vi "Lab Panel V4.91.vi"() -> ()   [LabVIEW 2013] (continued)
                                (unwired) FALSE
                                n567 = String To Path(string=w889) -> (path=w885:path)
                                n568 = TDMS Open(6:FALSE, 10:T20."create or replace" ("operation (0:open)"), 11:w885) -> (0:w884:errorcluster, 3:→"TDMS LAB01-2":refnum<k34>)  [unwired: 4 in]
                              }
                              frame #2 {
                                n569 = local read "SET LAB01-2"() -> (w895:T5)
                                n570 = local read "TDMS LAB01-2"() -> (w906:refnum<k34>)
                                n571 = Build Array("Testers Name", "Description", "Set Test Cycles", "T-Rise minutes", "T-Rise Deg C") -> (w896:string[])
                                n572 = Unbundle(w895) -> ("NAME"=w894:string, "DESCRIPTION"=w893:string, "CYCLES"=w892:dbl, "T-RISE mins"=w891:dbl, "T-RISE deg C"=w890:dbl)
                                n573 = Number To Decimal String(number=w892) -> (decimal integer string=w905:string)  [unwired: 1 in]
                                n574 = Number To Decimal String(number=w891) -> (decimal integer string=w904:string)  [unwired: 1 in]
                                n575 = Number To Decimal String(number=w890) -> (decimal integer string=w903:string)  [unwired: 1 in]
                                n576 = Build Array(w894, w893, w905, w904, w903) -> (w902:string[])
                                n577 = TDMS Set Properties(5:w902, 7:w896, 11:w906) -> ()  [unwired: 3 in, 4 out]
                              }
                              frame #3 {
                                n578 = local read "DISP LAB01-2"() -> (w908:T4)
                                n579 = Concatenate Strings("LAB01-2  ", w911) -> (w912:string)
                                n580 = Two Button Dialog(message=w912, 1:w909, 2:w910) -> (T button?=w914:bool)
                                n581 = case shown="True" w914 {
                                tunnel: w908 -> [w921 w922]
                                tunnel: [w921 w922] -> w918
                                tunnel: [w920 w923] -> w917
                                tunnel: [w919 w923] -> w916
                                frame False {
                                n582 = Unbundle(w921) -> ("CYCLE"=w920:dbl, "MINS"=w919:dbl)  [unwired: 1 out]
                                }
                                frame True {
                                w923 = 0.0
                                }
                                }
                                n583 = Bundle(cluster=w918, "CYCLE"=w917, "MINS"=w916, "STATUS"="RUN") -> (w907:T4)
                                n584 = local write "DISP LAB01-2"(w907) -> ()
                              }
                              frame #4 {
                                n585 = local read "TEMP START LAB01-2"() -> (w926:cluster{"TL":dbl, "TN":dbl})
                                n586 = Bundle(cluster=w926, "TL"=w924, "TN"=w924) -> (w925:cluster{"TL":dbl, "TN":dbl})
                                n587 = local write "TEMP START LAB01-2"(w925) -> ()
                              }
                            }
                          }
                        }
                      }
                    }
                  }
                }
              }
              event "RUN LAB02-1": Value Change {
                n588 = event-data() -> ("NewVal"=w932:bool)  [unwired: 1 in, 5 out]
                n589 = local read "SIG LAB02-1"() -> (w928:T2)
                n590 = case shown="True" w932 {
                  tunnel: w938 -> [_ w976]
                  tunnel: w937 -> [_ w975]
                  tunnel: w935 -> [w940 w974]
                  tunnel: w936 -> [_ w973]
                  tunnel: w934 -> [_ w972]
                  tunnel: [w939 w971] -> w933
                  tunnel: w931 -> [_ w970]
                  tunnel: w930 -> [_ w969]
                  tunnel: w929 -> [_ w968]
                  tunnel: w928 -> [_ w967]
                  tunnel: w927 -> [_ w966]
                  frame False {
                    # "stop test"
                    n591 = stacked-sequence {
                      tunnel: w940 -> [w949 _]
                      tunnel: [w941 _] -> w939
                      frame #0 {
                        n592 = local read "DISP LAB02-1"() -> (w948:T4)
                        n593 = Unbundle(w948) -> ("CYCLE"=w946:dbl, "MINS"=w947:dbl)  [unwired: 1 out]
                        n594 = case shown="\"CYCLE TEST\"" w949 {
                          tunnel: w947 -> [_ _ w956]
                          tunnel: w946 -> [w954 w955 _]
                          tunnel: [w954 w955 w956] -> w945
                          frame "CHART TEST", Default {
                          }
                          frame "CYCLE TEST" {
                          }
                          frame "T-RISE TEST" {
                          }
                        }
                        n595 = local read "TDMS LAB02-1"() -> (w953:refnum<k34>)
                        n596 = Build Array("STOPPED") -> (w950:string[])
                        n597 = Build Array(w945) -> (w944:dbl[])
                        n598 = TDMS Write(0:w953, 5:"TEST RESULT", 7:w950, 9:w944) -> (4:w942:refnum<k34>, 15:w943:errorcluster)  [unwired: 2 in, 2 out]
                        n599 = TDMS Close(8:w943, 11:w942) -> (0:w941:errorcluster)  [unwired: 1 out]
                      }
                      frame #1 {
                        n600 = local read "DISP LAB02-1"() -> (w960:T4)
                        n601 = stacked-sequence {
                          tunnel: "LAB02-1" -> [w962 w964]
                          frame #0 {
                            n602 = call "sub vi - defrag tdms v1.vi"("panel id"=w962) -> ("error out"=w961:errorcluster)  [unwired: 10 in]
                            n603 = local write "data file error"(w961) -> ()
                          }
                          frame #1 {
                            n604 = local write "RESULT LAB02-1"(FALSE) -> ()
                            n605 = call "Save data file (stop) v3.vi"("panel id"=w964) -> ("network file save error"=w963:errorcluster)  [unwired: 9 in, 1 out]
                            n606 = local write "data file error"(w963) -> ()
                          }
                        }
                        n607 = Bundle(cluster=w960, "STATUS"="STOP") -> (w958:T4)  [unwired: 2 in]
                        n608 = local write "DISP LAB02-1"(w958) -> ()
                      }
                    }
                  }
                  frame True {
                    n609 = stacked-sequence {
                      seq-local: [w978 _] -> [_ w982]
                      tunnel: w976 -> [_ w992]
                      tunnel: w975 -> [_ w991]
                      tunnel: w974 -> [_ w990]
                      tunnel: w973 -> [_ w989]
                      tunnel: w972 -> [_ w988]
                      tunnel: [_ w987] -> w971
                      tunnel: w970 -> [_ w986]
                      tunnel: w969 -> [_ w985]
                      tunnel: w968 -> [_ w984]
                      tunnel: w967 -> [w977 w983]
                      tunnel: w966 -> [_ w981]
                      frame #0 {
                        n610 = Unbundle(w977) -> ("AMPS"=w980:dbl)  [unwired: 4 out]
                        n611 = call "Check For Amps on v1.vi"("ID"="LAB02-1", "amps"=w980) -> ("amps"=w978:bool)  [unwired: 9 in]
                      }
                      frame #1 {
                        n612 = case shown="True" w982 {
                          tunnel: w992 -> [_ w1005]
                          tunnel: w991 -> [_ w1004]
                          tunnel: w990 -> [_ w1003]
                          tunnel: w989 -> [_ w1002]
                          tunnel: w988 -> [_ w1001]
                          tunnel: [errorcluster {"status"=FALSE, "code"=0, "source"=""} ("error out") w1000] -> w987
                          tunnel: w986 -> [_ w999]
                          tunnel: w985 -> [_ w998]
                          tunnel: w984 -> [_ w997]
                          tunnel: w983 -> [_ w996]
                          tunnel: w981 -> [_ w995]
                          frame False {
                            w994 = FALSE
                            n613 = local write "RUN LAB02-1"(w994) -> ()
                            n614 = local write "run lab02-1"(w994) -> ()
                          }
                          frame True {
                            n615 = stacked-sequence {
                              seq-local: [w1006 _ _ _ _] -> [_ w1030 _ _ _]
                              tunnel: w1005 -> [w1011 _ _ _ _]
                              tunnel: w1004 -> [w1008 _ _ _ _]
                              tunnel: w1003 -> [w1021 _ _ _ _]
                              tunnel: w1002 -> [w1014 _ _ _ _]
                              tunnel: w1001 -> [w1009 _ _ _ _]
                              tunnel: [_ w1025 _ _ _] -> w1000
                              tunnel: w999 -> [_ _ _ w1051 _]
                              tunnel: w998 -> [_ _ _ w1050 _]
                              tunnel: w997 -> [_ _ _ w1049 _]
                              tunnel: w996 -> [_ _ _ _ _]
                              tunnel: w995 -> [_ _ _ _ w1065]
                              frame #0 {
                                w1007 = "\\"
                                n616 = local read "SET LAB02-1"() -> (w1016:T5)
                                n617 = case shown="\"CYCLE TEST\"" w1021 {
                                tunnel: ["L02-1-CHART TEST-" "L02-1-CYCLE TEST-" "L02-1-T-RISE TEST-"] -> w1017
                                frame "CHART TEST", Default {
                                }
                                frame "CYCLE TEST" {
                                }
                                frame "T-RISE TEST" {
                                }
                                }
                                n618 = Unbundle(w1016) -> ("DESCRIPTION"=w1015:string)  [unwired: 4 out]
                                n619 = Concatenate Strings(w1011, "\\", w1009, w1007, w1008, w1007) -> (w1018:string)
                                n620 = String To Path(string=w1018) -> (path=w1020:path)
                                n621 = Concatenate Strings(w1018, w1017, w1015, "-", w1014, ".tdms") -> (w1006:string)
                                n622 = Create Folder(path (use dialog)=w1020) -> (error out=w1019:errorcluster)  [unwired: 2 in, 2 out]
                                n623 = global write "Global 1.vi" "LAB02-1 FILE"(w1006) -> ()
                                n624 = call <vilib>:"Clear Errors.vi"("error in (no error)"=w1019) -> ()  [unwired: 6 in, 1 out]
                              }
                              frame #1 {
                                (unwired) FALSE
                                n625 = String To Path(string=w1030) -> (path=w1026:path)
                                n626 = TDMS Open(6:FALSE, 10:T20."create or replace" ("operation (0:open)"), 11:w1026) -> (0:w1025:errorcluster, 3:→"TDMS LAB02-1":refnum<k34>)  [unwired: 4 in]
                              }
                              frame #2 {
                                n627 = local read "SET LAB02-1"() -> (w1036:T5)
                                n628 = local read "TDMS LAB02-1"() -> (w1047:refnum<k34>)
                                n629 = Build Array("Testers Name", "Description", "Set Test Cycles", "T-Rise minutes", "T-Rise Deg C") -> (w1037:string[])
                                n630 = Unbundle(w1036) -> ("NAME"=w1035:string, "DESCRIPTION"=w1034:string, "CYCLES"=w1033:dbl, "T-RISE mins"=w1032:dbl, "T-RISE deg C"=w1031:dbl)
                                n631 = Number To Decimal String(number=w1033) -> (decimal integer string=w1046:string)  [unwired: 1 in]
                                n632 = Number To Decimal String(number=w1032) -> (decimal integer string=w1045:string)  [unwired: 1 in]
                                n633 = Number To Decimal String(number=w1031) -> (decimal integer string=w1044:string)  [unwired: 1 in]
                                n634 = Build Array(w1035, w1034, w1046, w1045, w1044) -> (w1043:string[])
                                n635 = TDMS Set Properties(5:w1043, 7:w1037, 11:w1047) -> ()  [unwired: 3 in, 4 out]
                              }
                              frame #3 {
                                n636 = local read "DISP LAB02-1"() -> (w1052:T4)
                                n637 = Concatenate Strings("LAB02-1  ", w1051) -> (w1053:string)
                                n638 = Two Button Dialog(message=w1053, 1:w1049, 2:w1050) -> (T button?=w1055:bool)
                                n639 = case shown="True" w1055 {
                                tunnel: w1052 -> [w1062 w1063]
                                tunnel: [w1062 w1063] -> w1059
                                tunnel: [w1061 w1064] -> w1058
                                tunnel: [w1060 w1064] -> w1057
                                frame False {
                                n640 = Unbundle(w1062) -> ("CYCLE"=w1061:dbl, "MINS"=w1060:dbl)  [unwired: 1 out]
                                }
                                frame True {
                                w1064 = 0.0
                                }
                                }
                                n641 = Bundle(cluster=w1059, "CYCLE"=w1058, "MINS"=w1057, "STATUS"="RUN") -> (w1048:T4)
                                n642 = local write "DISP LAB02-1"(w1048) -> ()
                              }
                              frame #4 {
                                n643 = local read "TEMP START LAB02-1"() -> (w1067:cluster{"TL":dbl, "TN":dbl})
                                n644 = Bundle(cluster=w1067, "TL"=w1065, "TN"=w1065) -> (w1066:cluster{"TL":dbl, "TN":dbl})
                                n645 = local write "TEMP START LAB02-1"(w1066) -> ()
                              }
                            }
                          }
                        }
                      }
                    }
                  }
                }
                n646 = local write "run lab02-1"(w932) -> ()
              }
              event "RUN LAB02-2": Value Change {
                n647 = event-data() -> ("NewVal"=w1072:bool)  [unwired: 1 in, 5 out]
                n648 = local write "run lab02-2"(w1072) -> ()
                n649 = case shown="True" w1072 {
                  tunnel: w1078 -> [_ w1116]
                  tunnel: w1077 -> [_ w1115]
                  tunnel: w1075 -> [w1080 w1114]
                  tunnel: w1076 -> [_ w1113]
                  tunnel: w1074 -> [_ w1112]
                  tunnel: [w1079 w1111] -> w1073
                  tunnel: w1071 -> [_ w1110]
                  tunnel: w1070 -> [_ w1109]
                  tunnel: w1069 -> [_ w1108]
                  tunnel: w1068 -> [_ w1106]
                  frame False {
                    # "stop test"
                    n650 = stacked-sequence {
                      tunnel: w1080 -> [w1089 _]
                      tunnel: [w1081 _] -> w1079
                      frame #0 {
                        n651 = local read "DISP LAB02-2"() -> (w1088:T4)
                        n652 = Unbundle(w1088) -> ("CYCLE"=w1086:dbl, "MINS"=w1087:dbl)  [unwired: 1 out]
                        n653 = case shown="\"CYCLE TEST\"" w1089 {
                          tunnel: w1087 -> [_ _ w1096]
                          tunnel: w1086 -> [w1094 w1095 _]
                          tunnel: [w1094 w1095 w1096] -> w1085
                          frame "CHART TEST", Default {
                          }
                          frame "CYCLE TEST" {
                          }
                          frame "T-RISE TEST" {
                          }
                        }
                        n654 = local read "TDMS LAB02-2"() -> (w1093:refnum<k34>)
                        n655 = Build Array("STOPPED") -> (w1090:string[])
                        n656 = Build Array(w1085) -> (w1084:dbl[])
                        n657 = TDMS Write(0:w1093, 5:"TEST RESULT", 7:w1090, 9:w1084) -> (4:w1082:refnum<k34>, 15:w1083:errorcluster)  [unwired: 2 in, 2 out]
                        n658 = TDMS Close(8:w1083, 11:w1082) -> (0:w1081:errorcluster)  [unwired: 1 out]
                      }
                      frame #1 {
                        n659 = local read "DISP LAB02-2"() -> (w1100:T4)
                        n660 = stacked-sequence {
                          tunnel: "LAB02-2" -> [w1102 w1104]
                          frame #0 {
                            n661 = call "sub vi - defrag tdms v1.vi"("panel id"=w1102) -> ("error out"=w1101:errorcluster)  [unwired: 10 in]
                            n662 = local write "data file error"(w1101) -> ()
                          }
                          frame #1 {
                            n663 = call "Save data file (stop) v3.vi"("panel id"=w1104) -> ("network file save error"=w1103:errorcluster)  [unwired: 9 in, 1 out]
                            n664 = local write "RESULT LAB02-2"(FALSE) -> ()
                            n665 = local write "data file error"(w1103) -> ()
                          }
                        }
                        n666 = Bundle(cluster=w1100, "STATUS"="STOP") -> (w1098:T4)  [unwired: 2 in]
                        n667 = local write "DISP LAB02-2"(w1098) -> ()
                      }
                    }
                  }
                  frame True {
                    n668 = local read "SIG LAB02-2"() -> (w1107:T2)
                    n669 = stacked-sequence {
                      seq-local: [w1118 _] -> [_ w1122]
                      tunnel: w1116 -> [_ w1132]
                      tunnel: w1115 -> [_ w1131]
                      tunnel: w1114 -> [_ w1130]
                      tunnel: w1113 -> [_ w1129]
                      tunnel: w1112 -> [_ w1128]
                      tunnel: [_ w1127] -> w1111
                      tunnel: w1110 -> [_ w1126]
                      tunnel: w1109 -> [_ w1125]
                      tunnel: w1108 -> [_ w1124]
                      tunnel: w1107 -> [w1117 w1123]
                      tunnel: w1106 -> [_ w1121]
                      frame #0 {
                        n670 = Unbundle(w1117) -> ("AMPS"=w1120:dbl)  [unwired: 4 out]
                        n671 = call "Check For Amps on v1.vi"("ID"="LAB02-2", "amps"=w1120) -> ("amps"=w1118:bool)  [unwired: 9 in]
                      }
                      frame #1 {
                        n672 = case shown="True" w1122 {
                          tunnel: w1132 -> [_ w1145]
                          tunnel: w1131 -> [_ w1144]
                          tunnel: w1130 -> [_ w1143]
                          tunnel: w1129 -> [_ w1142]
                          tunnel: w1128 -> [_ w1141]
                          tunnel: [errorcluster {"status"=FALSE, "code"=0, "source"=""} ("error out") w1140] -> w1127
                          tunnel: w1126 -> [_ w1139]
                          tunnel: w1125 -> [_ w1138]
                          tunnel: w1124 -> [_ w1137]
                          tunnel: w1123 -> [_ w1136]
                          tunnel: w1121 -> [_ w1135]
                          frame False {
                            w1133 = FALSE
                            n673 = local write "RUN LAB02-2"(w1133) -> ()
                            n674 = local write "run lab02-2"(w1133) -> ()
                          }
                          frame True {
                            n675 = stacked-sequence {
                              seq-local: [w1146 _ _ _ _] -> [_ w1170 _ _ _]
                              tunnel: w1145 -> [w1151 _ _ _ _]
                              tunnel: w1144 -> [w1148 _ _ _ _]
                              tunnel: w1143 -> [w1161 _ _ _ _]
                              tunnel: w1142 -> [w1154 _ _ _ _]
                              tunnel: w1141 -> [w1149 _ _ _ _]
                              tunnel: [_ w1165 _ _ _] -> w1140
                              tunnel: w1139 -> [_ _ _ w1191 _]
                              tunnel: w1138 -> [_ _ _ w1190 _]
                              tunnel: w1137 -> [_ _ _ w1189 _]
                              tunnel: w1136 -> [_ _ _ _ _]
                              tunnel: w1135 -> [_ _ _ _ w1205]
                              frame #0 {
                                w1147 = "\\"
                                n676 = local read "SET LAB02-2"() -> (w1156:T5)
                                n677 = case shown="\"CYCLE TEST\"" w1161 {
                                tunnel: ["L02-2-CHART TEST-" "L02-2-CYCLE TEST-" "L02-2-T-RISE TEST-"] -> w1157
                                frame "CHART TEST", Default {
                                }
                                frame "CYCLE TEST" {
                                }
                                frame "T-RISE TEST" {
                                }
                                }
                                n678 = Unbundle(w1156) -> ("DESCRIPTION"=w1155:string)  [unwired: 4 out]
                                n679 = Concatenate Strings(w1151, "\\", w1149, w1147, w1148, w1147) -> (w1158:string)
                                n680 = String To Path(string=w1158) -> (path=w1160:path)
                                n681 = Concatenate Strings(w1158, w1157, w1155, "-", w1154, ".tdms") -> (w1146:string)
                                n682 = Create Folder(path (use dialog)=w1160) -> (error out=w1159:errorcluster)  [unwired: 2 in, 2 out]
                                n683 = global write "Global 1.vi" "LAB02-2 FILE"(w1146) -> ()
                                n684 = call <vilib>:"Clear Errors.vi"("error in (no error)"=w1159) -> ()  [unwired: 6 in, 1 out]
                              }
                              frame #1 {
                                (unwired) FALSE
                                n685 = String To Path(string=w1170) -> (path=w1166:path)
                                n686 = TDMS Open(6:FALSE, 10:T20."create or replace" ("operation (0:open)"), 11:w1166) -> (0:w1165:errorcluster, 3:→"TDMS LAB02-2":refnum<k34>)  [unwired: 4 in]
                              }
                              frame #2 {
                                n687 = local read "SET LAB02-2"() -> (w1176:T5)
                                n688 = local read "TDMS LAB02-2"() -> (w1187:refnum<k34>)
                                n689 = Build Array("Testers Name", "Description", "Set Test Cycles", "T-Rise minutes", "T-Rise Deg C") -> (w1177:string[])
                                n690 = Unbundle(w1176) -> ("NAME"=w1175:string, "DESCRIPTION"=w1174:string, "CYCLES"=w1173:dbl, "T-RISE mins"=w1172:dbl, "T-RISE deg C"=w1171:dbl)
                                n691 = Number To Decimal String(number=w1173) -> (decimal integer string=w1186:string)  [unwired: 1 in]
                                n692 = Number To Decimal String(number=w1172) -> (decimal integer string=w1185:string)  [unwired: 1 in]
                                n693 = Number To Decimal String(number=w1171) -> (decimal integer string=w1184:string)  [unwired: 1 in]
                                n694 = Build Array(w1175, w1174, w1186, w1185, w1184) -> (w1183:string[])
                                n695 = TDMS Set Properties(5:w1183, 7:w1177, 11:w1187) -> ()  [unwired: 3 in, 4 out]
                              }
                              frame #3 {
                                n696 = local read "DISP LAB02-2"() -> (w1192:T4)
                                n697 = Concatenate Strings("LAB02-2  ", w1191) -> (w1193:string)
                                n698 = Two Button Dialog(message=w1193, 1:w1189, 2:w1190) -> (T button?=w1195:bool)
                                n699 = case shown="True" w1195 {
                                tunnel: w1192 -> [w1202 w1203]
                                tunnel: [w1202 w1203] -> w1199
                                tunnel: [w1201 w1204] -> w1198
                                tunnel: [w1200 w1204] -> w1197
                                frame False {
                                n700 = Unbundle(w1202) -> ("CYCLE"=w1201:dbl, "MINS"=w1200:dbl)  [unwired: 1 out]
                                }
                                frame True {
                                w1204 = 0.0
                                }
                                }
                                n701 = Bundle(cluster=w1199, "CYCLE"=w1198, "MINS"=w1197, "STATUS"="RUN") -> (w1188:T4)
                                n702 = local write "DISP LAB02-2"(w1188) -> ()
                              }
                              frame #4 {
                                n703 = local read "TEMP START LAB02-2"() -> (w1207:cluster{"TL":dbl, "TN":dbl})
                                n704 = Bundle(cluster=w1207, "TL"=w1205, "TN"=w1205) -> (w1206:cluster{"TL":dbl, "TN":dbl})
                                n705 = local write "TEMP START LAB02-2"(w1206) -> ()
                              }
                            }
                          }
                        }
                      }
                    }
                  }
                }
              }
              event "RUN LAB03-1": Value Change {
                n706 = event-data() -> ("NewVal"=w1212:bool)  [unwired: 1 in, 5 out]
                n707 = local write "run lab03-1"(w1212) -> ()
                n708 = case shown="True" w1212 {
                  tunnel: w1218 -> [_ w1256]
                  tunnel: w1217 -> [_ w1255]
                  tunnel: w1215 -> [w1220 w1254]
                  tunnel: w1216 -> [_ w1253]
                  tunnel: w1214 -> [_ w1252]
                  tunnel: [w1219 w1251] -> w1213
                  tunnel: w1211 -> [_ w1250]
                  tunnel: w1210 -> [_ w1249]
                  tunnel: w1209 -> [_ w1248]
                  tunnel: w1208 -> [_ w1246]
                  frame False {
                    # "stop test"
                    n709 = stacked-sequence {
                      tunnel: w1220 -> [w1229 _]
                      tunnel: [w1221 _] -> w1219
                      frame #0 {
                        n710 = local read "DISP LAB03-1"() -> (w1228:T4)
                        n711 = Unbundle(w1228) -> ("CYCLE"=w1226:dbl, "MINS"=w1227:dbl)  [unwired: 1 out]
                        n712 = case shown="\"CYCLE TEST\"" w1229 {
                          tunnel: w1227 -> [_ _ w1236]
                          tunnel: w1226 -> [w1234 w1235 _]
                          tunnel: [w1234 w1235 w1236] -> w1225
                          frame "CHART TEST", Default {
                          }
                          frame "CYCLE TEST" {
                          }
                          frame "T-RISE TEST" {
                          }
                        }
                        n713 = local read "TDMS LAB03-1"() -> (w1233:refnum<k34>)
                        n714 = Build Array("STOPPED") -> (w1230:string[])
                        n715 = Build Array(w1225) -> (w1224:dbl[])
                        n716 = TDMS Write(0:w1233, 5:"TEST RESULT", 7:w1230, 9:w1224) -> (4:w1222:refnum<k34>, 15:w1223:errorcluster)  [unwired: 2 in, 2 out]
                        n717 = TDMS Close(8:w1223, 11:w1222) -> (0:w1221:errorcluster)  [unwired: 1 out]
                      }
                      frame #1 {
                        n718 = local read "DISP LAB03-1"() -> (w1240:T4)
                        n719 = stacked-sequence {
                          tunnel: "LAB03-1" -> [w1242 w1244]
                          frame #0 {
                            n720 = call "sub vi - defrag tdms v1.vi"("panel id"=w1242) -> ("error out"=w1241:errorcluster)  [unwired: 10 in]
                            n721 = local write "data file error"(w1241) -> ()
                          }
                          frame #1 {
                            n722 = call "Save data file (stop) v3.vi"("panel id"=w1244) -> ("network file save error"=w1243:errorcluster)  [unwired: 9 in, 1 out]
                            n723 = local write "RESULT LAB03-1"(FALSE) -> ()
                            n724 = local write "data file error"(w1243) -> ()
                          }
                        }
                        n725 = Bundle(cluster=w1240, "STATUS"="STOP") -> (w1238:T4)  [unwired: 2 in]
                        n726 = local write "DISP LAB03-1"(w1238) -> ()
                      }
                    }
                  }
                  frame True {
                    n727 = local read "SIG LAB03-1"() -> (w1247:T2)
                    n728 = stacked-sequence {
                      seq-local: [w1258 _] -> [_ w1262]
                      tunnel: w1256 -> [_ w1272]
                      tunnel: w1255 -> [_ w1271]
                      tunnel: w1254 -> [_ w1270]
                      tunnel: w1253 -> [_ w1269]
                      tunnel: w1252 -> [_ w1268]
                      tunnel: [_ w1267] -> w1251
                      tunnel: w1250 -> [_ w1266]
                      tunnel: w1249 -> [_ w1265]
                      tunnel: w1248 -> [_ w1264]
                      tunnel: w1247 -> [w1257 w1263]
                      tunnel: w1246 -> [_ w1261]
                      frame #0 {
                        n729 = Unbundle(w1257) -> ("AMPS"=w1260:dbl)  [unwired: 4 out]
                        n730 = call "Check For Amps on v1.vi"("ID"="LAB03-1", "amps"=w1260) -> ("amps"=w1258:bool)  [unwired: 9 in]
                      }
                      frame #1 {
                        n731 = case shown="True" w1262 {
                          tunnel: w1272 -> [_ w1285]
                          tunnel: w1271 -> [_ w1284]
                          tunnel: w1270 -> [_ w1283]
                          tunnel: w1269 -> [_ w1282]
                          tunnel: w1268 -> [_ w1281]
                          tunnel: [errorcluster {"status"=FALSE, "code"=0, "source"=""} ("error out") w1280] -> w1267
                          tunnel: w1266 -> [_ w1279]
                          tunnel: w1265 -> [_ w1278]
                          tunnel: w1264 -> [_ w1277]
                          tunnel: w1263 -> [_ w1276]
                          tunnel: w1261 -> [_ w1275]
                          frame False {
                            w1273 = FALSE
                            n732 = local write "RUN LAB03-1"(w1273) -> ()
                            n733 = local write "run lab03-1"(w1273) -> ()
                          }
                          frame True {
                            n734 = stacked-sequence {
                              seq-local: [w1286 _ _ _ _] -> [_ w1310 _ _ _]
                              tunnel: w1285 -> [w1291 _ _ _ _]
                              tunnel: w1284 -> [w1288 _ _ _ _]
                              tunnel: w1283 -> [w1301 _ _ _ _]
                              tunnel: w1282 -> [w1294 _ _ _ _]
                              tunnel: w1281 -> [w1289 _ _ _ _]
                              tunnel: [_ w1305 _ _ _] -> w1280
                              tunnel: w1279 -> [_ _ _ w1330 _]
                              tunnel: w1278 -> [_ _ _ w1329 _]
                              tunnel: w1277 -> [_ _ _ w1328 _]
                              tunnel: w1276 -> [_ _ _ _ _]
                              tunnel: w1275 -> [_ _ _ _ w1345]
                              frame #0 {
                                w1287 = "\\"
                                n735 = local read "SET LAB03-1"() -> (w1296:T5)
                                n736 = case shown="\"T-RISE TEST\"" w1301 {
                                tunnel: ["L03-1-CHART TEST-" "L03-1-CYCLE TEST-" "L03-1-T-RISE TEST-"] -> w1297
                                frame "CHART TEST", Default {
                                }
                                frame "CYCLE TEST" {
                                }
                                frame "T-RISE TEST" {
                                }
                                }
                                n737 = Unbundle(w1296) -> ("DESCRIPTION"=w1295:string)  [unwired: 4 out]
                                n738 = Concatenate Strings(w1291, "\\", w1289, w1287, w1288, w1287) -> (w1298:string)
                                n739 = String To Path(string=w1298) -> (path=w1300:path)
                                n740 = Concatenate Strings(w1298, w1297, w1295, "-", w1294, ".tdms") -> (w1286:string)
                                n741 = Create Folder(path (use dialog)=w1300) -> (error out=w1299:errorcluster)  [unwired: 2 in, 2 out]
                                n742 = global write "Global 1.vi" "LAB03-1 FILE"(w1286) -> ()
                                n743 = call <vilib>:"Clear Errors.vi"("error in (no error)"=w1299) -> ()  [unwired: 6 in, 1 out]
                              }
                              frame #1 {
                                (unwired) FALSE
                                n744 = String To Path(string=w1310) -> (path=w1306:path)
                                n745 = TDMS Open(6:FALSE, 10:T20."create or replace" ("operation (0:open)"), 11:w1306) -> (0:w1305:errorcluster, 3:→"TDMS LAB03-1":refnum<k34>)  [unwired: 4 in]
                              }
                              frame #2 {
                                n746 = local read "SET LAB03-1"() -> (w1316:T5)
                                n747 = local read "TDMS LAB03-1"() -> (w1327:refnum<k34>)
                                n748 = Build Array("Testers Name", "Description", "Set Test Cycles", "T-Rise minutes", "T-Rise Deg C") -> (w1317:string[])
                                n749 = Unbundle(w1316) -> ("NAME"=w1315:string, "DESCRIPTION"=w1314:string, "CYCLES"=w1313:dbl, "T-RISE mins"=w1312:dbl, "T-RISE deg C"=w1311:dbl)
                                n750 = Number To Decimal String(number=w1313) -> (decimal integer string=w1326:string)  [unwired: 1 in]
                                n751 = Number To Decimal String(number=w1312) -> (decimal integer string=w1325:string)  [unwired: 1 in]
                                n752 = Number To Decimal String(number=w1311) -> (decimal integer string=w1324:string)  [unwired: 1 in]
                                n753 = Build Array(w1315, w1314, w1326, w1325, w1324) -> (w1323:string[])
                                n754 = TDMS Set Properties(5:w1323, 7:w1317, 11:w1327) -> ()  [unwired: 3 in, 4 out]
                              }
                              frame #3 {
                                n755 = local read "DISP LAB03-1"() -> (w1332:T4)
                                n756 = Concatenate Strings("LAB03-1  ", w1330) -> (w1333:string)
                                n757 = Two Button Dialog(message=w1333, 1:w1328, 2:w1329) -> (T button?=w1335:bool)
                                n758 = case shown="True" w1335 {
                                tunnel: w1332 -> [w1342 w1343]
                                tunnel: [w1342 w1343] -> w1339
                                tunnel: [w1341 w1344] -> w1338
                                tunnel: [w1340 w1344] -> w1337
                                frame False {
                                n759 = Unbundle(w1342) -> ("CYCLE"=w1341:dbl, "MINS"=w1340:dbl)  [unwired: 1 out]
                                }
                                frame True {
                                w1344 = 0.0
                                }
                                }
                                n760 = Bundle(cluster=w1339, "CYCLE"=w1338, "MINS"=w1337, "STATUS"="RUN") -> (w1331:T4)
                                n761 = local write "DISP LAB03-1"(w1331) -> ()
                              }
                              frame #4 {
                                n762 = local read "TEMP START LAB03-1"() -> (w1347:cluster{"TL":dbl, "TN":dbl})
                                n763 = Bundle(cluster=w1347, "TL"=w1345, "TN"=w1345) -> (w1346:cluster{"TL":dbl, "TN":dbl})
                                n764 = local write "TEMP START LAB03-1"(w1346) -> ()
                              }
                            }
                          }
                        }
                      }
                    }
                  }
                }
              }
              event "RUN LAB03-2": Value Change {
                n765 = event-data() -> ("NewVal"=w1352:bool)  [unwired: 1 in, 5 out]
                n766 = local write "run lab03-2"(w1352) -> ()
                n767 = case shown="True" w1352 {
                  tunnel: w1358 -> [_ w1396]
                  tunnel: w1357 -> [_ w1395]
                  tunnel: w1355 -> [w1360 w1394]
                  tunnel: w1356 -> [_ w1393]
                  tunnel: w1354 -> [_ w1392]
                  tunnel: [w1359 w1391] -> w1353
                  tunnel: w1351 -> [_ w1390]
                  tunnel: w1350 -> [_ w1389]
                  tunnel: w1349 -> [_ w1388]
                  tunnel: w1348 -> [_ w1386]
                  frame False {
                    # "stop test"
                    n768 = stacked-sequence {
                      tunnel: w1360 -> [w1369 _]
                      tunnel: [w1361 _] -> w1359
                      frame #0 {
                        n769 = local read "DISP LAB03-2"() -> (w1368:T4)
                        n770 = Unbundle(w1368) -> ("CYCLE"=w1366:dbl, "MINS"=w1367:dbl)  [unwired: 1 out]
                        n771 = case shown="\"CYCLE TEST\"" w1369 {
                          tunnel: w1367 -> [_ _ w1376]
                          tunnel: w1366 -> [w1374 w1375 _]
                          tunnel: [w1374 w1375 w1376] -> w1365
                          frame "CHART TEST", Default {
                          }
                          frame "CYCLE TEST" {
                          }
                          frame "T-RISE TEST" {
                          }
                        }
                        n772 = local read "TDMS LAB03-2"() -> (w1373:refnum<k34>)
                        n773 = Build Array("STOPPED") -> (w1370:string[])
                        n774 = Build Array(w1365) -> (w1364:dbl[])
                        n775 = TDMS Write(0:w1373, 5:"TEST RESULT", 7:w1370, 9:w1364) -> (4:w1362:refnum<k34>, 15:w1363:errorcluster)  [unwired: 2 in, 2 out]
                        n776 = TDMS Close(8:w1363, 11:w1362) -> (0:w1361:errorcluster)  [unwired: 1 out]
                      }
                      frame #1 {
                        n777 = local read "DISP LAB03-2"() -> (w1380:T4)
                        n778 = stacked-sequence {
                          tunnel: "LAB03-2" -> [w1382 w1384]
                          frame #0 {
                            n779 = call "sub vi - defrag tdms v1.vi"("panel id"=w1382) -> ("error out"=w1381:errorcluster)  [unwired: 10 in]
                            n780 = local write "data file error"(w1381) -> ()
                          }
                          frame #1 {
                            n781 = call "Save data file (stop) v3.vi"("panel id"=w1384) -> ("network file save error"=w1383:errorcluster)  [unwired: 9 in, 1 out]
                            n782 = local write "RESULT LAB03-2"(FALSE) -> ()
                            n783 = local write "data file error"(w1383) -> ()
                          }
                        }
                        n784 = Bundle(cluster=w1380, "STATUS"="STOP") -> (w1378:T4)  [unwired: 2 in]
                        n785 = local write "DISP LAB03-2"(w1378) -> ()
                      }
                    }
                  }
                  frame True {
                    n786 = local read "SIG LAB03-2"() -> (w1387:T2)
                    n787 = stacked-sequence {
                      seq-local: [w1398 _] -> [_ w1402]
                      tunnel: w1396 -> [_ w1412]
                      tunnel: w1395 -> [_ w1411]
                      tunnel: w1394 -> [_ w1410]
                      tunnel: w1393 -> [_ w1409]
                      tunnel: w1392 -> [_ w1408]
                      tunnel: [_ w1407] -> w1391
                      tunnel: w1390 -> [_ w1406]
                      tunnel: w1389 -> [_ w1405]
                      tunnel: w1388 -> [_ w1404]
                      tunnel: w1387 -> [w1397 w1403]
                      tunnel: w1386 -> [_ w1401]
                      frame #0 {
                        n788 = Unbundle(w1397) -> ("AMPS"=w1400:dbl)  [unwired: 4 out]
                        n789 = call "Check For Amps on v1.vi"("ID"="LAB03-2", "amps"=w1400) -> ("amps"=w1398:bool)  [unwired: 9 in]
                      }
                      frame #1 {
                        n790 = case shown="True" w1402 {
                          tunnel: w1412 -> [_ w1425]
                          tunnel: w1411 -> [_ w1424]
                          tunnel: w1410 -> [_ w1423]
                          tunnel: w1409 -> [_ w1422]
                          tunnel: w1408 -> [_ w1421]
                          tunnel: [errorcluster {"status"=FALSE, "code"=0, "source"=""} ("error out") w1420] -> w1407
                          tunnel: w1406 -> [_ w1419]
                          tunnel: w1405 -> [_ w1418]
                          tunnel: w1404 -> [_ w1417]
                          tunnel: w1403 -> [_ w1416]
                          tunnel: w1401 -> [_ w1415]
                          frame False {
                            w1413 = FALSE
                            n791 = local write "RUN LAB03-2"(w1413) -> ()
                            n792 = local write "run lab03-2"(w1413) -> ()
                          }
                          frame True {
                            n793 = stacked-sequence {
                              seq-local: [w1426 _ _ _ _] -> [_ w1450 _ _ _]
                              tunnel: w1425 -> [w1431 _ _ _ _]
                              tunnel: w1424 -> [w1428 _ _ _ _]
                              tunnel: w1423 -> [w1441 _ _ _ _]
                              tunnel: w1422 -> [w1434 _ _ _ _]
                              tunnel: w1421 -> [w1429 _ _ _ _]
                              tunnel: [_ w1445 _ _ _] -> w1420
                              tunnel: w1419 -> [_ _ _ w1471 _]
                              tunnel: w1418 -> [_ _ _ w1470 _]
                              tunnel: w1417 -> [_ _ _ w1469 _]
                              tunnel: w1416 -> [_ _ _ _ _]
                              tunnel: w1415 -> [_ _ _ _ w1485]
                              frame #0 {
                                w1427 = "\\"
                                n794 = local read "SET LAB03-2"() -> (w1436:T5)
                                n795 = case shown="\"T-RISE TEST\"" w1441 {
                                tunnel: ["L03-2-CHART TEST-" "L03-2-CYCLE TEST-" "L03-2-T-RISE TEST-"] -> w1437
                                frame "CHART TEST", Default {
                                }
                                frame "CYCLE TEST" {
                                }
                                frame "T-RISE TEST" {
                                }
                                }
                                n796 = Unbundle(w1436) -> ("DESCRIPTION"=w1435:string)  [unwired: 4 out]
                                n797 = Concatenate Strings(w1431, "\\", w1429, w1427, w1428, w1427) -> (w1438:string)
                                n798 = String To Path(string=w1438) -> (path=w1440:path)
                                n799 = Concatenate Strings(w1438, w1437, w1435, "-", w1434, ".tdms") -> (w1426:string)
                                n800 = Create Folder(path (use dialog)=w1440) -> (error out=w1439:errorcluster)  [unwired: 2 in, 2 out]
                                n801 = global write "Global 1.vi" "LAB03-2 FILE"(w1426) -> ()
                                n802 = call <vilib>:"Clear Errors.vi"("error in (no error)"=w1439) -> ()  [unwired: 6 in, 1 out]
                              }
                              frame #1 {
                                (unwired) FALSE
                                n803 = String To Path(string=w1450) -> (path=w1446:path)
                                n804 = TDMS Open(6:FALSE, 10:T20."create or replace" ("operation (0:open)"), 11:w1446) -> (0:w1445:errorcluster, 3:→"TDMS LAB03-2":refnum<k34>)  [unwired: 4 in]
                              }
                              frame #2 {
                                n805 = local read "SET LAB03-2"() -> (w1456:T5)
                                n806 = local read "TDMS LAB03-2"() -> (w1467:refnum<k34>)
                                n807 = Build Array("Testers Name", "Description", "Set Test Cycles", "T-Rise minutes", "T-Rise Deg C") -> (w1457:string[])
                                n808 = Unbundle(w1456) -> ("NAME"=w1455:string, "DESCRIPTION"=w1454:string, "CYCLES"=w1453:dbl, "T-RISE mins"=w1452:dbl, "T-RISE deg C"=w1451:dbl)
                                n809 = Number To Decimal String(number=w1453) -> (decimal integer string=w1466:string)  [unwired: 1 in]
                                n810 = Number To Decimal String(number=w1452) -> (decimal integer string=w1465:string)  [unwired: 1 in]
                                n811 = Number To Decimal String(number=w1451) -> (decimal integer string=w1464:string)  [unwired: 1 in]
                                n812 = Build Array(w1455, w1454, w1466, w1465, w1464) -> (w1463:string[])
                                n813 = TDMS Set Properties(5:w1463, 7:w1457, 11:w1467) -> ()  [unwired: 3 in, 4 out]
                              }
                              frame #3 {
                                n814 = local read "DISP LAB03-2"() -> (w1472:T4)
                                n815 = Concatenate Strings("LAB03-2  ", w1471) -> (w1473:string)
                                n816 = Two Button Dialog(message=w1473, 1:w1469, 2:w1470) -> (T button?=w1475:bool)
                                n817 = case shown="True" w1475 {
                                tunnel: w1472 -> [w1482 w1483]
                                tunnel: [w1482 w1483] -> w1479
                                tunnel: [w1481 w1484] -> w1478
                                tunnel: [w1480 w1484] -> w1477
                                frame False {
                                n818 = Unbundle(w1482) -> ("CYCLE"=w1481:dbl, "MINS"=w1480:dbl)  [unwired: 1 out]
                                }
                                frame True {
                                w1484 = 0.0
                                }
                                }
                                n819 = Bundle(cluster=w1479, "CYCLE"=w1478, "MINS"=w1477, "STATUS"="RUN") -> (w1468:T4)
                                n820 = local write "DISP LAB03-2"(w1468) -> ()
                              }
                              frame #4 {
                                n821 = local read "TEMP START LAB03-2"() -> (w1487:cluster{"TL":dbl, "TN":dbl})
                                n822 = Bundle(cluster=w1487, "TL"=w1485, "TN"=w1485) -> (w1486:cluster{"TL":dbl, "TN":dbl})
                                n823 = local write "TEMP START LAB03-2"(w1486) -> ()
                              }
                            }
                          }
                        }
                      }
                    }
                  }
                }
              }
              event "RUN LAB04-1": Value Change {
                n824 = event-data() -> ("NewVal"=w1492:bool)  [unwired: 1 in, 5 out]
                n825 = local write "run lab04-1"(w1492) -> ()
                n826 = case shown="True" w1492 {
                  tunnel: w1498 -> [_ w1536]
                  tunnel: w1497 -> [_ w1535]
                  tunnel: w1495 -> [w1500 w1534]
                  tunnel: w1496 -> [_ w1533]
                  tunnel: w1494 -> [_ w1532]
                  tunnel: [w1499 w1531] -> w1493
                  tunnel: w1491 -> [_ w1530]
                  tunnel: w1490 -> [_ w1529]
                  tunnel: w1489 -> [_ w1528]
                  tunnel: w1488 -> [_ w1526]
                  frame False {
                    # "stop test"
                    n827 = stacked-sequence {
                      tunnel: w1500 -> [w1509 _]
                      tunnel: [w1501 _] -> w1499
                      frame #0 {
                        n828 = local read "DISP LAB04-1"() -> (w1508:T4)
                        n829 = Unbundle(w1508) -> ("CYCLE"=w1506:dbl, "MINS"=w1507:dbl)  [unwired: 1 out]
                        n830 = case shown="\"CYCLE TEST\"" w1509 {
                          tunnel: w1507 -> [_ _ w1516]
                          tunnel: w1506 -> [w1514 w1515 _]
                          tunnel: [w1514 w1515 w1516] -> w1505
                          frame "CHART TEST", Default {
                          }
                          frame "CYCLE TEST" {
                          }
                          frame "T-RISE TEST" {
                          }
                        }
                        n831 = local read "TDMS LAB04-1"() -> (w1513:refnum<k34>)
                        n832 = Build Array("STOPPED") -> (w1510:string[])
                        n833 = Build Array(w1505) -> (w1504:dbl[])
                        n834 = TDMS Write(0:w1513, 5:"TEST RESULT", 7:w1510, 9:w1504) -> (4:w1502:refnum<k34>, 15:w1503:errorcluster)  [unwired: 2 in, 2 out]
                        n835 = TDMS Close(8:w1503, 11:w1502) -> (0:w1501:errorcluster)  [unwired: 1 out]
                      }
                      frame #1 {
                        n836 = local read "DISP LAB04-1"() -> (w1520:T4)
                        n837 = stacked-sequence {
                          tunnel: "LAB04-1" -> [w1522 w1524]
                          frame #0 {
                            n838 = call "sub vi - defrag tdms v1.vi"("panel id"=w1522) -> ("error out"=w1521:errorcluster)  [unwired: 10 in]
                            n839 = local write "data file error"(w1521) -> ()
                          }
                          frame #1 {
